vi "TimeoutDelay_example.vi"   [LabVIEW 2014]
uses:
  <vilib>/Aledyne-TSXperts/Arduino Compatible Compiler for LabVIEW/Code Generator/Arduino APIs/Digital/PinDirection.ctl
  QwaveSys_ESP8266/QwaveSys_ESP8266.lvlib
  <vilib>/Aledyne-TSXperts/Arduino Compatible Compiler for LabVIEW/Arduino Compatible Compiler for LabVIEW.lvlib
types:
  T1 = typedef "Arduino Compatible Compiler for LabVIEW.lvlib/PinDirection.ctl" = enum16{" INPUT", "OUTPUT", " INPUT_PULLUP"}
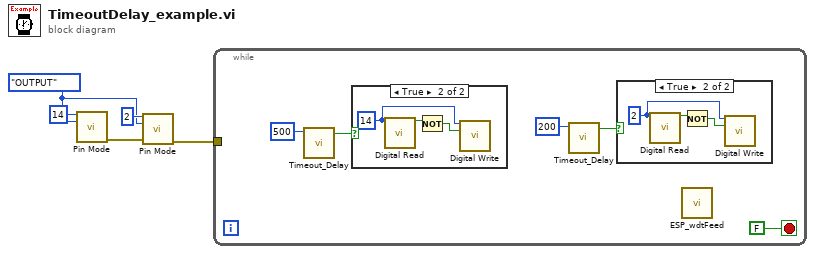
[diagram p0: block diagram]
diagram:
  w2 = PinDirection."OUTPUT" ("direction")
  n1 = call <vilib>:"Pin Mode.vi"("pin"=u8 14, "direction"=w2) -> ("error out"=w4:errorcluster)  [unwired: 13 in]
  n2 = call <vilib>:"Pin Mode.vi"("pin"=u8 2, "direction"=w2, "error in (no error)"=w4) -> ("error out"=w1:errorcluster)  [unwired: 12 in]
  n3 = while {
    tunnel: w1 -> [_]
    stop <- FALSE stop-if-true
    n4 = call "Timeout_Delay.vi"("timeout (ms)"=u32 500) -> ("status"=w8:bool)  [unwired: 8 in, 2 out]
    n5 = case shown="True" w8 {
      frame False {
      }
      frame True {
        w14 = u8 14 ("pin")
        n6 = call <vilib>:"Digital Read.vi"("pin"=w14) -> ("state"=w16:bool)  [unwired: 13 in, 1 out]
        n7 = Not(x=w16) -> (.not. x?=w15:bool)
        n8 = call <vilib>:"Digital Write.vi"("pin"=w14, "state"=w15) -> ()  [unwired: 13 in, 1 out]
      }
    }
    n9 = call "Timeout_Delay.vi"("timeout (ms)"=u32 200) -> ("status"=w7:bool)  [unwired: 8 in, 2 out]
    n10 = case shown="True" w7 {
      frame False {
      }
      frame True {
        w11 = u8 2 ("pin")
        n11 = call <vilib>:"Digital Read.vi"("pin"=w11) -> ("state"=w13:bool)  [unwired: 13 in, 1 out]
        n12 = Not(x=w13) -> (.not. x?=w12:bool)
        n13 = call <vilib>:"Digital Write.vi"("pin"=w11, "state"=w12) -> ()  [unwired: 13 in, 1 out]
      }
    }
    n14 = call "ESP_wdtFeed.vi"() -> ()  [unwired: 11 in, 1 out]
  }
